vi "To JSON.vi"(8 "error in (no error)":errorcluster, 10 "Anything":variant) -> (0 "error out":errorcluster, 2 "JSON":string)   [LabVIEW 2017, in "Transparent Assertions.lvlib"]
uses:
  <vilib>/PNR/JSONtext Object Serialization/Generic Object Serializer/Generic Object Serializer.lvclass
  C:/Program Files/National Instruments/LabVIEW 2017/vi.lib/JDP Science/JSONtext/LVClass Serializer/JSONtext LVClass Serializer.lvclass
  c34f3794-71bb-4fc1-98c1-2c7c55f09150.vi
  <vilib>/JDP Science/JSONtext/Variant to JSON Text.vi
  Transparent Assertions.lvlib
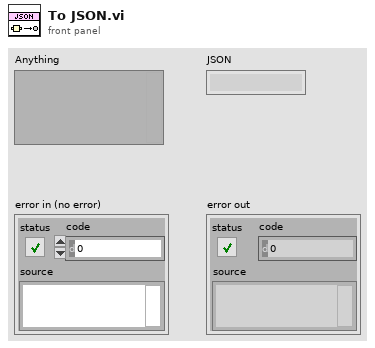
[diagram p1: front panel]
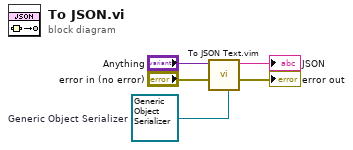
[diagram p0: block diagram]
diagram:
  w1 = refnum<class "Generic Object Serializer.lvclass"> refnum  # Generic Object Serializer
  n1 = call "To JSON Text.vim"("LVClass Serializer"=w1, "error in (no error)"="error in (no error)", "Anything"="Anything") -> ("error out"=→"error out":errorcluster, "<JSON>"=→"JSON":string)  [unwired: 7 in]
